vi "CODmn启动器.vi"(11 "控制命令":enum16{"水样测试", "平行样测试", "加标回收", "停止"}(ring)) -> ()   [LabVIEW 2016, in "质控单元V4.lvlib"]
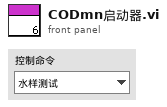
[diagram p1: front panel]
types:
  T1 = cluster{"测量模式":enum16{"水样测量", "标样核查", "零点核查", "跨度核查", "空白测试", "加标回收", "平行样", "校零", "校标"}}
  T2 = cluster{"站号":u16, "量程切换":enum32{"H", "L", "AUTO"}, "控制命令":enum16{"启动测量", "标样核查", "零点核查", "跨度核查", "空白测试", "平行样测试", "加标回收", "空白校准", "标样校准", "初始化（清洗）", "停止测试", "仪器重启", "校时", "模式设置", "测量间隔设置"}, "模式设置":enum16{"待机", "连续模式", "周期模式", "定点模式", "受控模式", "手动模式"}, "测量间隔":u16}
  T3 = enum16{"启动测量", "标样核查", "零点核查", "跨度核查", "空白测试", "平行样测试", "加标回收", "空白校准", "标样校准", "初始化（清洗）", "停止测试", "仪器重启", "校时", "模式设置", "测量间隔设置"}
  T4 = cluster{"水样测试量程模式":enum16{"H", "L", "AUTO"}, "空白核查量程模式":enum16{"H", "L", "AUTO"}, "跨度核查量程模式":enum16{"H", "L", "AUTO"}, "加标回收量程模式":enum16{"H", "L", "AUTO"}}
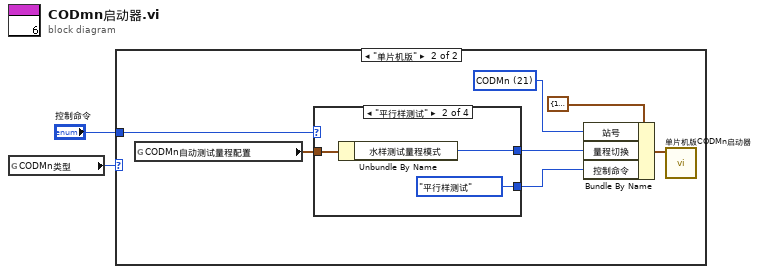
[diagram p0: block diagram]
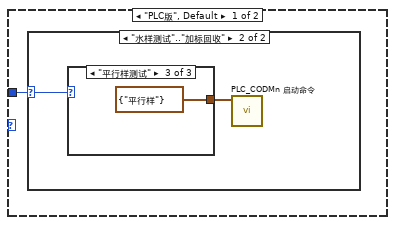
[diagram p2: hidden frame]
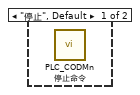
[diagram p3: hidden frame]
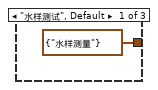
[diagram p4: hidden frame]
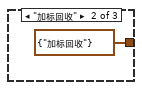
[diagram p5: hidden frame]
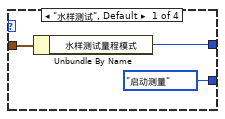
[diagram p6: hidden frame]
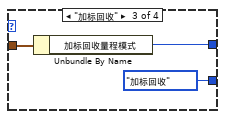
[diagram p7: hidden frame]
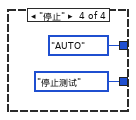
[diagram p8: hidden frame]
diagram:
  n1 = global read "系统交互.vi" "CODMn类型"() -> (w2:enum16{"PLC版", "单片机版"})
  n2 = case shown="\"单片机版\"" w2 {
    tunnel: "控制命令" -> [w3 w13]
    frame "PLC版", Default {
      n3 = case shown="\"水样测试\"..\"加标回收\"" w3 {
        selector: w3 -> [_ w5]
        frame "停止", Default {
          n4 = call "PLC_CODMn 停止命令.vi"() -> ()  [unwired: 12 in]
        }
        frame "水样测试".."加标回收" {
          n5 = case shown="\"平行样测试\"" w5 {
            tunnel: [T1 {"测量模式"=enum."水样测量"} ("启动测量模式") T1 {"测量模式"=enum."加标回收"} ("启动测量模式") T1 {"测量模式"=enum."平行样"} ("启动测量模式")] -> w4
            frame "水样测试", Default {
            }
            frame "加标回收" {
            }
            frame "平行样测试" {
            }
          }
          n6 = call "PLC_CODMn 启动命令.vi"("启动测量模式"=w4) -> ()  [unwired: 11 in]
        }
      }
    }
    frame "单片机版" {
      w15 = u16 21 items=["总磷"=1, "总氮"=2, "氨氮"=3, "CODMn"=21] ("站号")
      n7 = global read "系统交互.vi" "CODMn自动测试量程配置"() -> (w12:T4)
      n8 = case shown="\"平行样测试\"" w13 {
        tunnel: [T3."启动测量" T3."平行样测试" T3."加标回收" T3."停止测试"] -> w11
        tunnel: w12 -> [w17 w20 w23 _]
        tunnel: [w16 w19 w22 enum16{"H", "L", "AUTO"}."AUTO" ("加标回收量程模式")] -> w10
        frame "水样测试", Default {
          n9 = Unbundle By Name(w17) -> ("水样测试量程模式"=w16:enum16{"H", "L", "AUTO"})
        }
        frame "平行样测试" {
          n10 = Unbundle By Name(w20) -> ("水样测试量程模式"=w19:enum16{"H", "L", "AUTO"})
        }
        frame "加标回收" {
          n11 = Unbundle By Name(w23) -> ("加标回收量程模式"=w22:enum16{"H", "L", "AUTO"})
        }
        frame "停止" {
        }
      }
      n12 = Bundle By Name(cluster=T2 {"站号"=1, "量程切换"=enum."AUTO", "控制命令"=enum."启动测量", "模式设置"=enum."待机", "测量间隔"=0} ("参数"), "站号"=w15, "量程切换"=w10, "控制命令"=w11) -> (w9:T2)
      n13 = call "单片机版CODMn启动器.vi"("参数"=w9) -> ()  [unwired: 10 in, 1 out]
    }
  }
